vi "CheckBeginScore.vi"(0 "object in":refnum<class "StandardAttackPlay.lvclass">, 3 "GameRef":refnum<data-value>, 5 "error in (no error)":errorcluster) -> (14 "object out":refnum<class "StandardAttackPlay.lvclass">, 16 "score":dbl, 19 "error out":errorcluster)   [LabVIEW 2023, in "StandardAttackPlay.lvclass"]
uses:
  StandardAttackPlay.lvclass
  Game_class/Game.lvclass
  Play_v2_class/Play_v2.lvclass
  StandardAttackPlay.lvclass/StandardAttackPlay.ctl
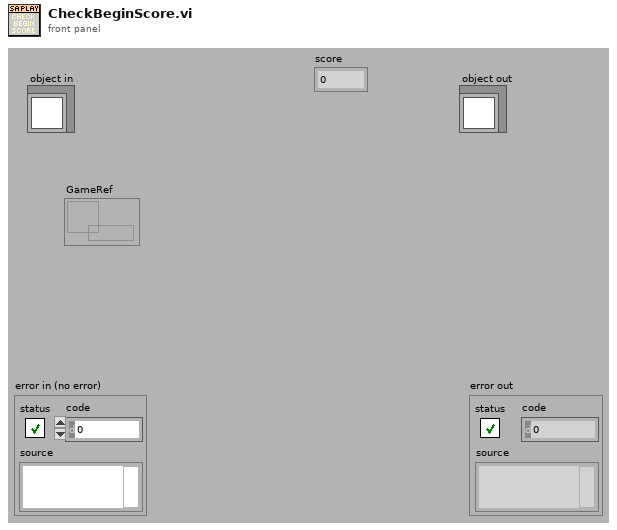
[diagram p1: front panel]
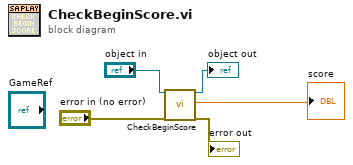
[diagram p0: block diagram]
diagram:
  n1 = call-parent "CheckBeginScore.vi"("object in"="object in", "error in (no error)"="error in (no error)") -> ("object out"=→"object out":refnum<class "StandardAttackPlay.lvclass">, "score"=→"score":dbl, "error out"=→"error out":errorcluster)  [unwired: 15 in]
